vi "dMSE_dOut.vi"(9 "Data inputs":sgl, 10 "Label (expected output":sgl, 11 "Output":sgl) -> (3 "Numeric":sgl)   [LabVIEW 2020]
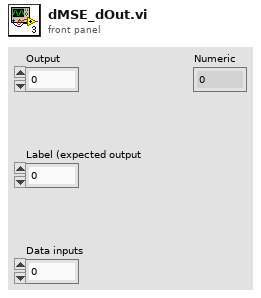
[diagram p1: front panel]
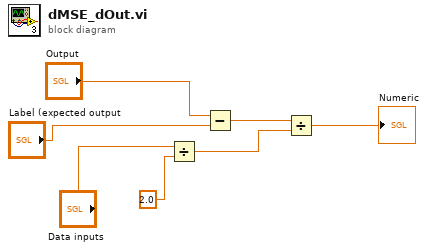
[diagram p0: block diagram]
diagram:
  n1 = Divide(x="Data inputs", y=sgl 2.0) -> (x/y=w7:sgl)
  n2 = Subtract(x="Output", y="Label (expected output") -> (x-y=w2:sgl)
  n3 = Divide(x=w2, y=w7) -> (x/y=→"Numeric":sgl)
